vi "OverwriteSingleParameter.vi"(9 "MainConfigurationArrayIN":cluster{"Parameter":string, "Value":string}[](array[cluster]), 10 "Value":string, 11 "Parameter":string) -> (1 "MainConfigurationArrayOUT":cluster{"Parameter":string, "Value":string}[](array[cluster]))   [LabVIEW 2017]
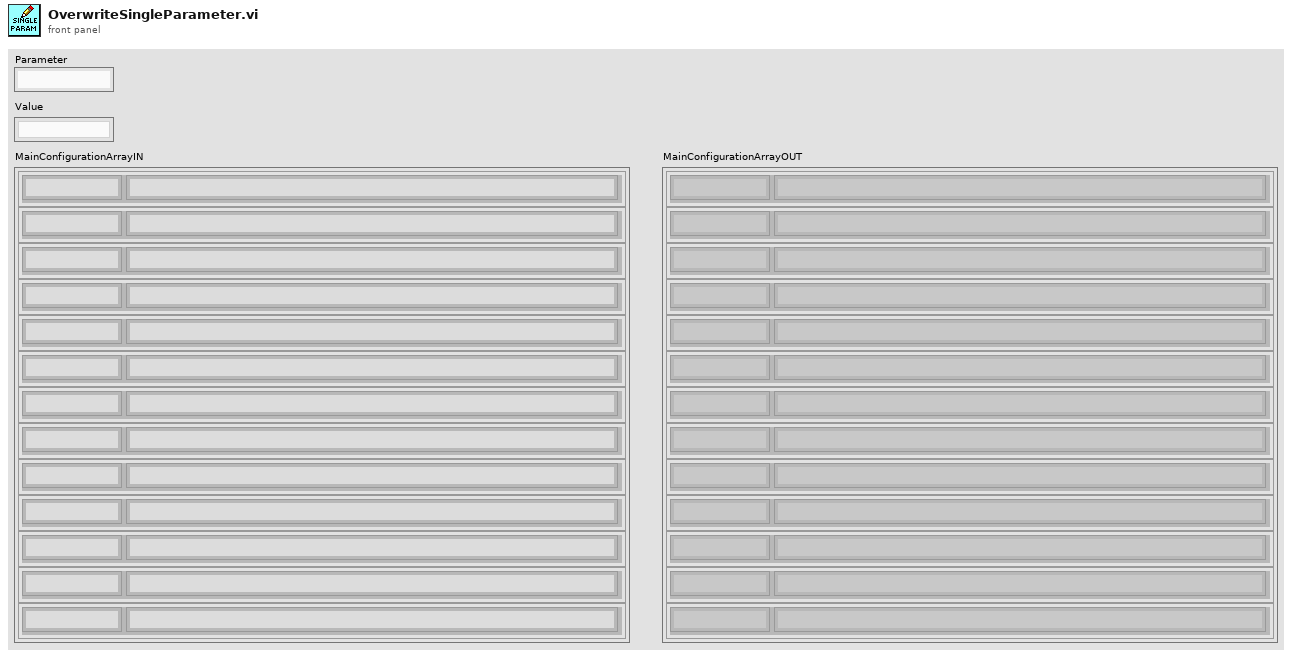
[diagram p1: front panel]
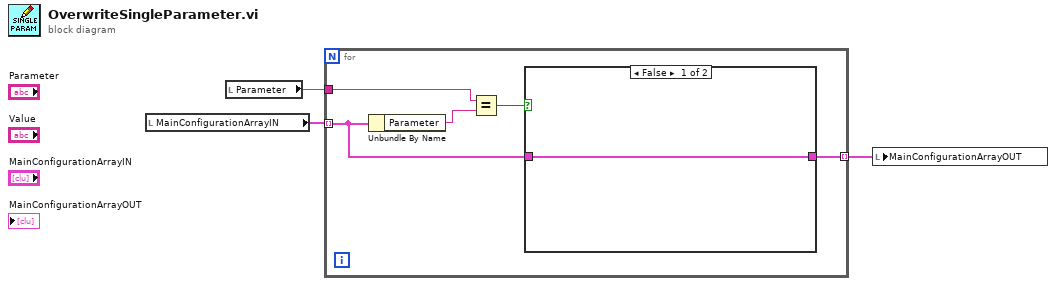
[diagram p0: block diagram]
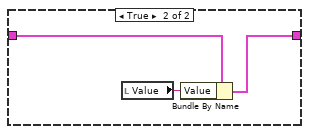
[diagram p2: hidden frame]
diagram:
  n1 = local read "MainConfigurationArrayIN"() -> (w2:cluster{"Parameter":string, "Value":string}[])
  n2 = local read "Parameter"() -> (w3:string)
  n3 = for {
    tunnel: w2 -> [w5] mode=indexing
    tunnel: w3 -> [w7]
    tunnel: [w4] -> w1 mode=indexing
    n4 = Unbundle By Name(w5) -> ("Parameter"=w8:string)
    n5 = Equal?(x=w7, y=w8) -> (x = y?=w6:bool)
    n6 = case shown="False" w6 {
      tunnel: w5 -> [w9 w11]
      tunnel: [w9 w10] -> w4
      frame False {
      }
      frame True {
        n7 = local read "Value"() -> (w12:string)
        n8 = Bundle By Name(cluster=w11, "Value"=w12) -> (w10:cluster{"Parameter":string, "Value":string})
      }
    }
  }
  n9 = local write "MainConfigurationArrayOUT"(w1) -> ()
